vi "Split PV and Field Names.vi"(2 "default field":string="value", 3 "PV name / field":string) -> (0 "field name":string, 1 "PV name":string)   [LabVIEW 2020, in "PV Access.lvlib"]
doc: "Wire a string to <B>PV name / field</B> like \"my:pv/timeStamp/nanoseconds\" then <B>PV name</B> will be \"my:pv\" and <B>field name</B> will be \"timeStamp.nanoseconds\".\n\nIf no field is appended the PV name then the <B>default field</B> will be used."
uses:
  PV Access.lvlib
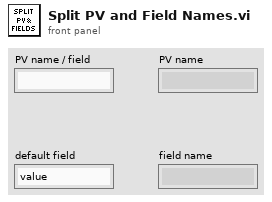
[diagram p1: front panel]
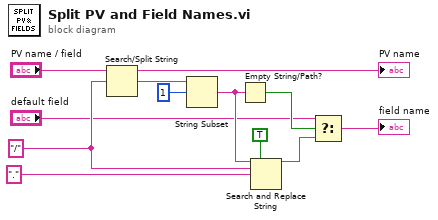
[diagram p0: block diagram]
diagram:
  w4 = "/" ("search string/char (-)")
  n1 = Search/Split String(string="PV name / field", search string/char (-)=w4) -> (substring before match=→"PV name":string, match + rest of string=w12:string)  [unwired: 1 in, 1 out]
  n2 = String Subset(string=w12, offset (0)=1) -> (substring=w6:string)  [unwired: 1 in]
  n3 = Empty String/Path?(string/path=w6) -> (empty?=w10:bool)
  n4 = Search and Replace String(replace all?=TRUE ("replace all? (F)"), input string=w6, search string=w4, replace string="." ("replace string (\"\")")) -> (result string=w2:string)  [unwired: 4 in, 3 out]
  n5 = Select(t="default field", s=w10, f=w2) -> (s? t:f=→"field name":string)
